vi "Init.vi"(3 "Container State":T4, 4 "Previous State":variant, 5 "Previous Version":T3) -> (2 "Current State":T1)   [LabVIEW 2015, in "Noise (G3).xctl"]
uses:
  Noise (G3).xctl
  State.ctl
  Noise (G3) - Persistent.ctl
  <vilib>/_xctls/Container State.ctl
  <vilib>/_xctls/Version.ctl
  <vilib>/_xctls/XControlSupport.lvlib
panel:
  in  "Default Indicator State":T1={"enable menu"=TRUE, "persistent"={"Show Aweight"=FALSE}}
  in  "Default Control State":T1={"enable menu"=TRUE, "persistent"={"Show Aweight"=FALSE}}
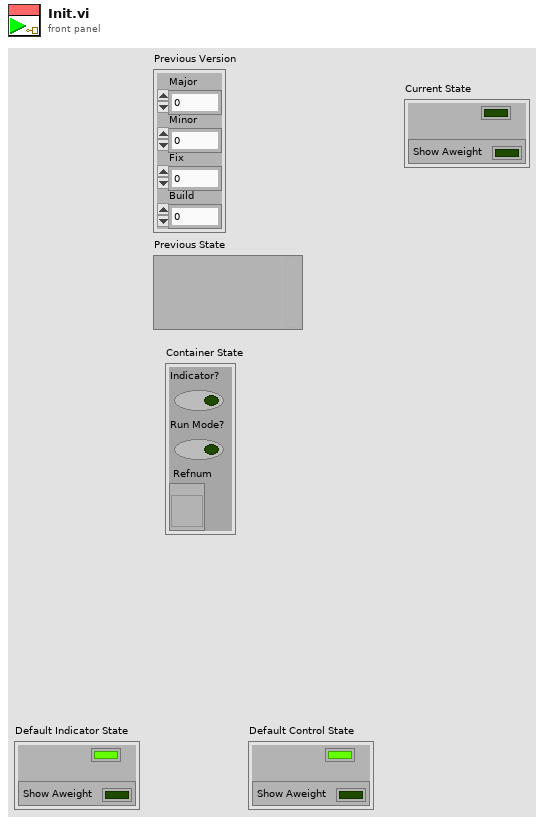
[diagram p1: front panel]
types:
  T1 = typedef "Noise (G3).xctl/State.ctl" = cluster{"enable menu":bool, "persistent":T2}
  T2 = typedef "Noise (G3).xctl/Noise (G3) - Persistent.ctl" = cluster{"Show Aweight":bool}
  T3 = typedef "XControlSupport.lvlib/Version.ctl" = cluster{"Major":u16, "Minor":u16, "Fix":u16, "Build":u16}
  T4 = typedef "XControlSupport.lvlib/Container State.ctl" = cluster{"Indicator?":bool, "Run Mode?":bool, " Refnum":refnum<vi>}
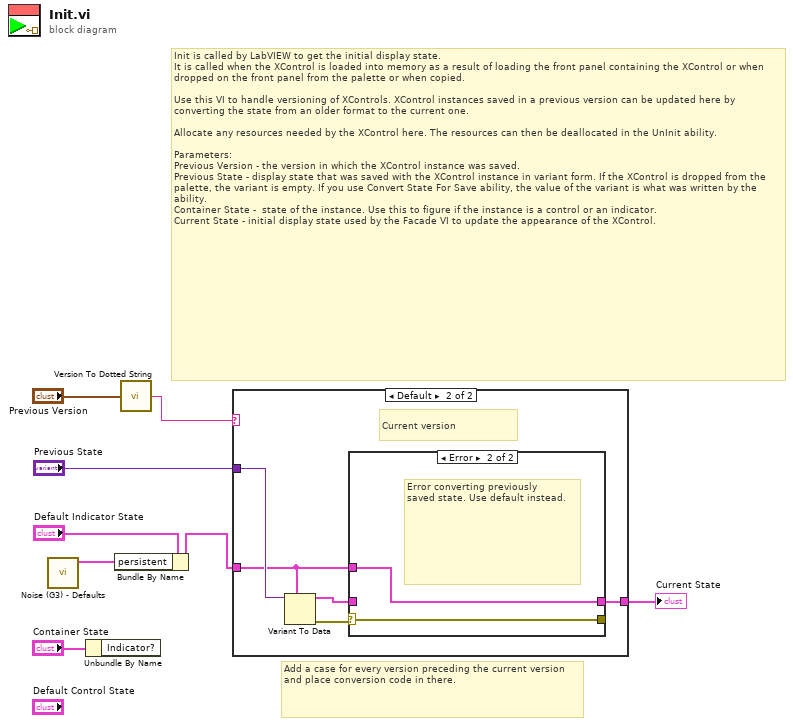
[diagram p0: block diagram]
diagram:
  # "Add a case for every version preceding the current version and place conversion code in there."
  # "Init is called by LabVIEW to get the initial display state.\nIt is called when the XControl is loaded into memory as a result of loading the front panel containing the XControl or when dropped on the front panel from the palette or when copied.\n\nUse this VI to handle versioning of XControls. XControl instances saved in a previous version can be updated here by converting the state from an older format to the current one.\n\nAllocate any resources needed by the XControl here. The resources can then be deallocated in the UnInit ability.\n\nParameters:\nPrevious Version - the version in which the XControl instance was saved.\nPrevious State - display state that was saved with the XControl instance in variant form. If the XControl is dropped from the palette, the variant is empty. If you use Convert State For Save ability, the value of the variant is what was written by the ability. \nContainer State -  state of the instance. Use this to figure if the instance is a control or an indicator.\nCurrent State - initial display state used by the Facade VI to update the appearance of the XControl."
  n1 = call "Noise (G3) - Defaults.vi"() -> ("persistent"=w2:T2)  [unwired: 11 in]
  n2 = Unbundle By Name("Container State") -> ()  [unwired: 1 out]
  n3 = Bundle By Name(cluster="Default Indicator State", "persistent"=w2) -> (w3:T1)
  n4 = call <vilib>:"Version To Dotted String.vi"("Version"="Previous Version") -> ("String Version"=w5:string)
  n5 = case shown="Default" w5 {
    tunnel: "Previous State" -> [_ w14]
    tunnel: [w9 w10] -> w1
    tunnel: w3 -> [w9 w11]
    frame "0.0.0.0" {
      # "Just created, use default state"
    }
    frame Default {
      # "Current version"
      n6 = Variant To Data(type=w11, Variant=w14) -> (data=w12:T1, error out=w13:errorcluster)  [unwired: 1 in]
      n7 = case shown="Error" w13 {
        selector: w13 -> [w16 w17]
        tunnel: w12 -> [w15 _]
        tunnel: [w15 w18] -> w10
        tunnel: w11 -> [_ w18]
        tunnel: [w16 w17] -> _
        frame No Error {
        }
        frame Error {
          # "Error converting previously \nsaved state. Use default instead."
        }
      }
    }
  }
  "Current State" <- w1
